vi "build.vi"(8 "error in (no error)":errorcluster, 11 "FrameBuilder in":refnum<class "FrameBuilder.lvclass">) -> (0 "error out":errorcluster, 2 "Frame":T1 {"Data" format="%02x"}, 3 "FrameBuilder out":refnum<class "FrameBuilder.lvclass">)   [LabVIEW 2015, in "RTModbus.lvlib" / "FrameBuilder.lvclass"]
uses:
  FrameBuilder.lvclass
  DataTypes/Frame.ctl
  FrameBuilder.lvclass/FrameBuilder.ctl
  RTModbus.lvlib
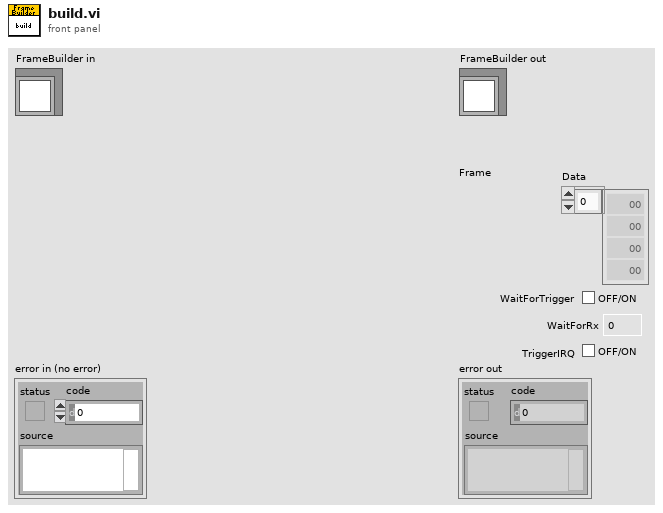
[diagram p1: front panel]
types:
  T1 = typedef "RTModbus.lvlib/Frame.ctl" = cluster{"Data":u8[], "WaitForTrigger":bool, "WaitForRx":u16, "TriggerIRQ":bool}
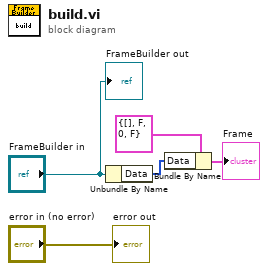
[diagram p0: block diagram]
diagram:
  n1 = Unbundle By Name("FrameBuilder in") -> ("Data"=w3:u8[])
  n2 = Bundle By Name(cluster=T1 {"Data"=[], "WaitForTrigger"=FALSE, "WaitForRx"=0, "TriggerIRQ"=FALSE} ("Frame"), "Data"=w3) -> (→"Frame":T1)
  "error out" <- "error in (no error)"
  "FrameBuilder out" <- "FrameBuilder in"
